vi "Configure IIC Trigger.vi"(5 "IIC Data (\"0x34XF\")":string="0x34XF", 6 "Address to Trigger (\"0x34XF\")":string="0x34XF", 7 "Trigger Type (0: Start)":i32(ring) items=["Start", "Stop", "Restart7", "Restart10", "Address ACK", "Address with No ACK", "Read7", "Write7", "Write10"], 8 "error in (no error)":errorcluster, 9 "Address Size (0: Bit7)":i32(ring) items=["Bit7", "Bit8"], 10 "Channel (1: Serial Bus 1)":i32(ring)=1 items=["Serial Bus 1"=1, "Serial Bus 2"=2, "Serial Bus 3"=3, "Serial Bus 4"=4], 11 "VISA resource name":refnum<visa-resource-name>) -> (0 "error out":errorcluster, 3 "VISA resource name out":refnum<visa-resource-name>)   [LabVIEW 2013, in "Agilent 90000 Series.lvlib"]
doc: "Configures IIC trigger settings.\n\n<B>Note:</B>\nThis VI is only valid when the low-speed IIC serial decode option has been licensed."
uses:
  Agilent 90000 Series.lvlib
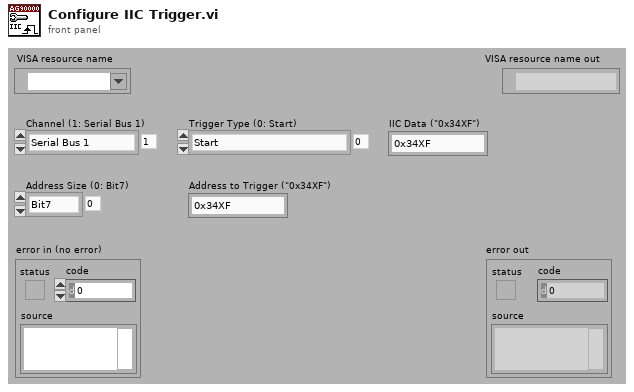
[diagram p1: front panel]
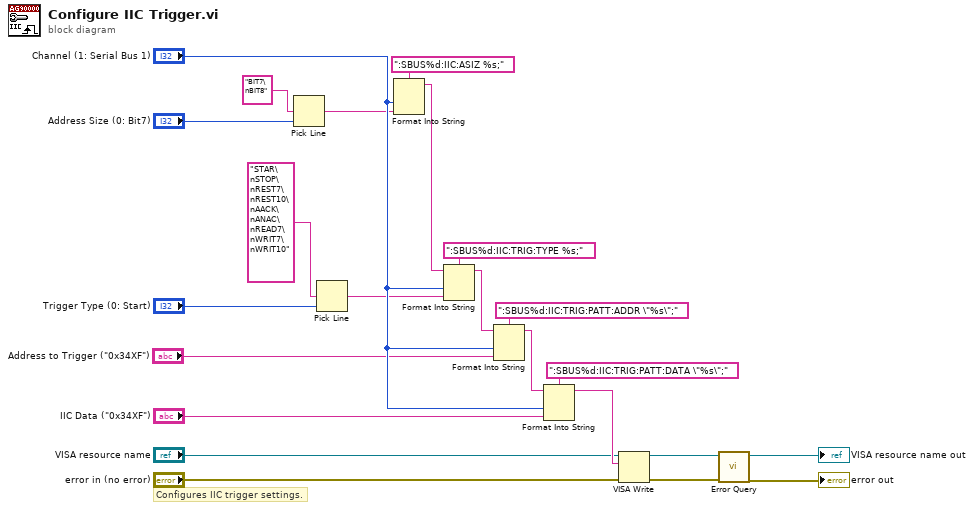
[diagram p0: block diagram]
diagram:
  # "Configures IIC trigger settings."
  n1 = Pick Line(multi-line string="BIT7\nBIT8", line index="Address Size (0: Bit7)") -> (output string=w19:string)  [unwired: 1 out]
  n2 = Pick Line(multi-line string="STAR\nSTOP\nREST7\nREST10\nAACK\nANAC\nREAD7\nWRIT7\nWRIT10", line index="Trigger Type (0: Start)") -> (output string=w14:string)  [unwired: 1 out]
  n3 = Format Into String(format string=":SBUS%d:IIC:ASIZ %s;", "Channel (1: Serial Bus 1)", w19) -> (resulting string=w16:string)  [unwired: 2 in, 1 out]
  n4 = Format Into String(format string=":SBUS%d:IIC:TRIG:TYPE %s;", initial string=w16, "Channel (1: Serial Bus 1)", w14) -> (resulting string=w13:string)  [unwired: 1 in, 1 out]
  n5 = Format Into String(format string=":SBUS%d:IIC:TRIG:PATT:ADDR \"%s\";", initial string=w13, "Channel (1: Serial Bus 1)", "Address to Trigger (\"0x34XF\")") -> (resulting string=w10:string)  [unwired: 1 in, 1 out]
  n6 = Format Into String(format string=":SBUS%d:IIC:TRIG:PATT:DATA \"%s\";", initial string=w10, "Channel (1: Serial Bus 1)", "IIC Data (\"0x34XF\")") -> (resulting string=w7:string)  [unwired: 1 in, 1 out]
  n7 = VISA Write(VISA resource name="VISA resource name", write buffer=w7, error in (no error)="error in (no error)") -> (VISA resource name out=w4:refnum<visa-resource-name>, error out=w3:errorcluster)  [unwired: 1 out]
  n8 = call "Error Query.vi"("error in (no error)"=w3, "VISA resource name"=w4) -> ("error out"=→"error out":errorcluster, "VISA resource name out"=→"VISA resource name out":refnum<visa-resource-name>)  [unwired: 8 out]
